vi "内部交互全局变量.vi"() -> ()   [LabVIEW 2016, in "环境动力监测库.lvlib"]
panel:
  out "监测配置输出":T1
  in  "名称或相对路径":string="data\\pem.ini"
  out "仁科通信解析":T2
  out "其他":T3 {"北斗-GPS"."GPS"."纬度:" format="%#.2g"; "北斗-GPS"."GPS"."经度:" format="%#.2g"; "北斗-GPS"."北斗"."纬度:" format="%#.2g"; "北斗-GPS"."北斗"."经度:" format="%#.2g"}
  out "安防模块":T4
  out "暖通模块":T5
  out "供电模块":T6 {"蓄电池24V"."电量" format="%.0f %"; "蓄电池24V"."电池电量:" scale=0.0..100.0; "蓄电池12V"."电量" format="%.0f %"; "蓄电池12V"."电池电量:" scale=0.0..100.0; "UPS"."电量" format="%.0f %"; "UPS"."电池电量:" scale=0.0..100.0}
  out "遥控开关机状态":bool
  out "系统参数":T7
  out "告警状态":T8
  out "传感器状态":T9
  out "运行状态":T10
  # "电源管理"
  # "GPS"
  # "北斗"
  # "真角"
  # "m/s"
  # "℃"
  # "bars"
  # "℃"
  # "℃"
  # "℃"
  # "V"
  # "V"
  # "V"
  # "V"
  # "V"
  # "V"
  # "A"
  # "V"
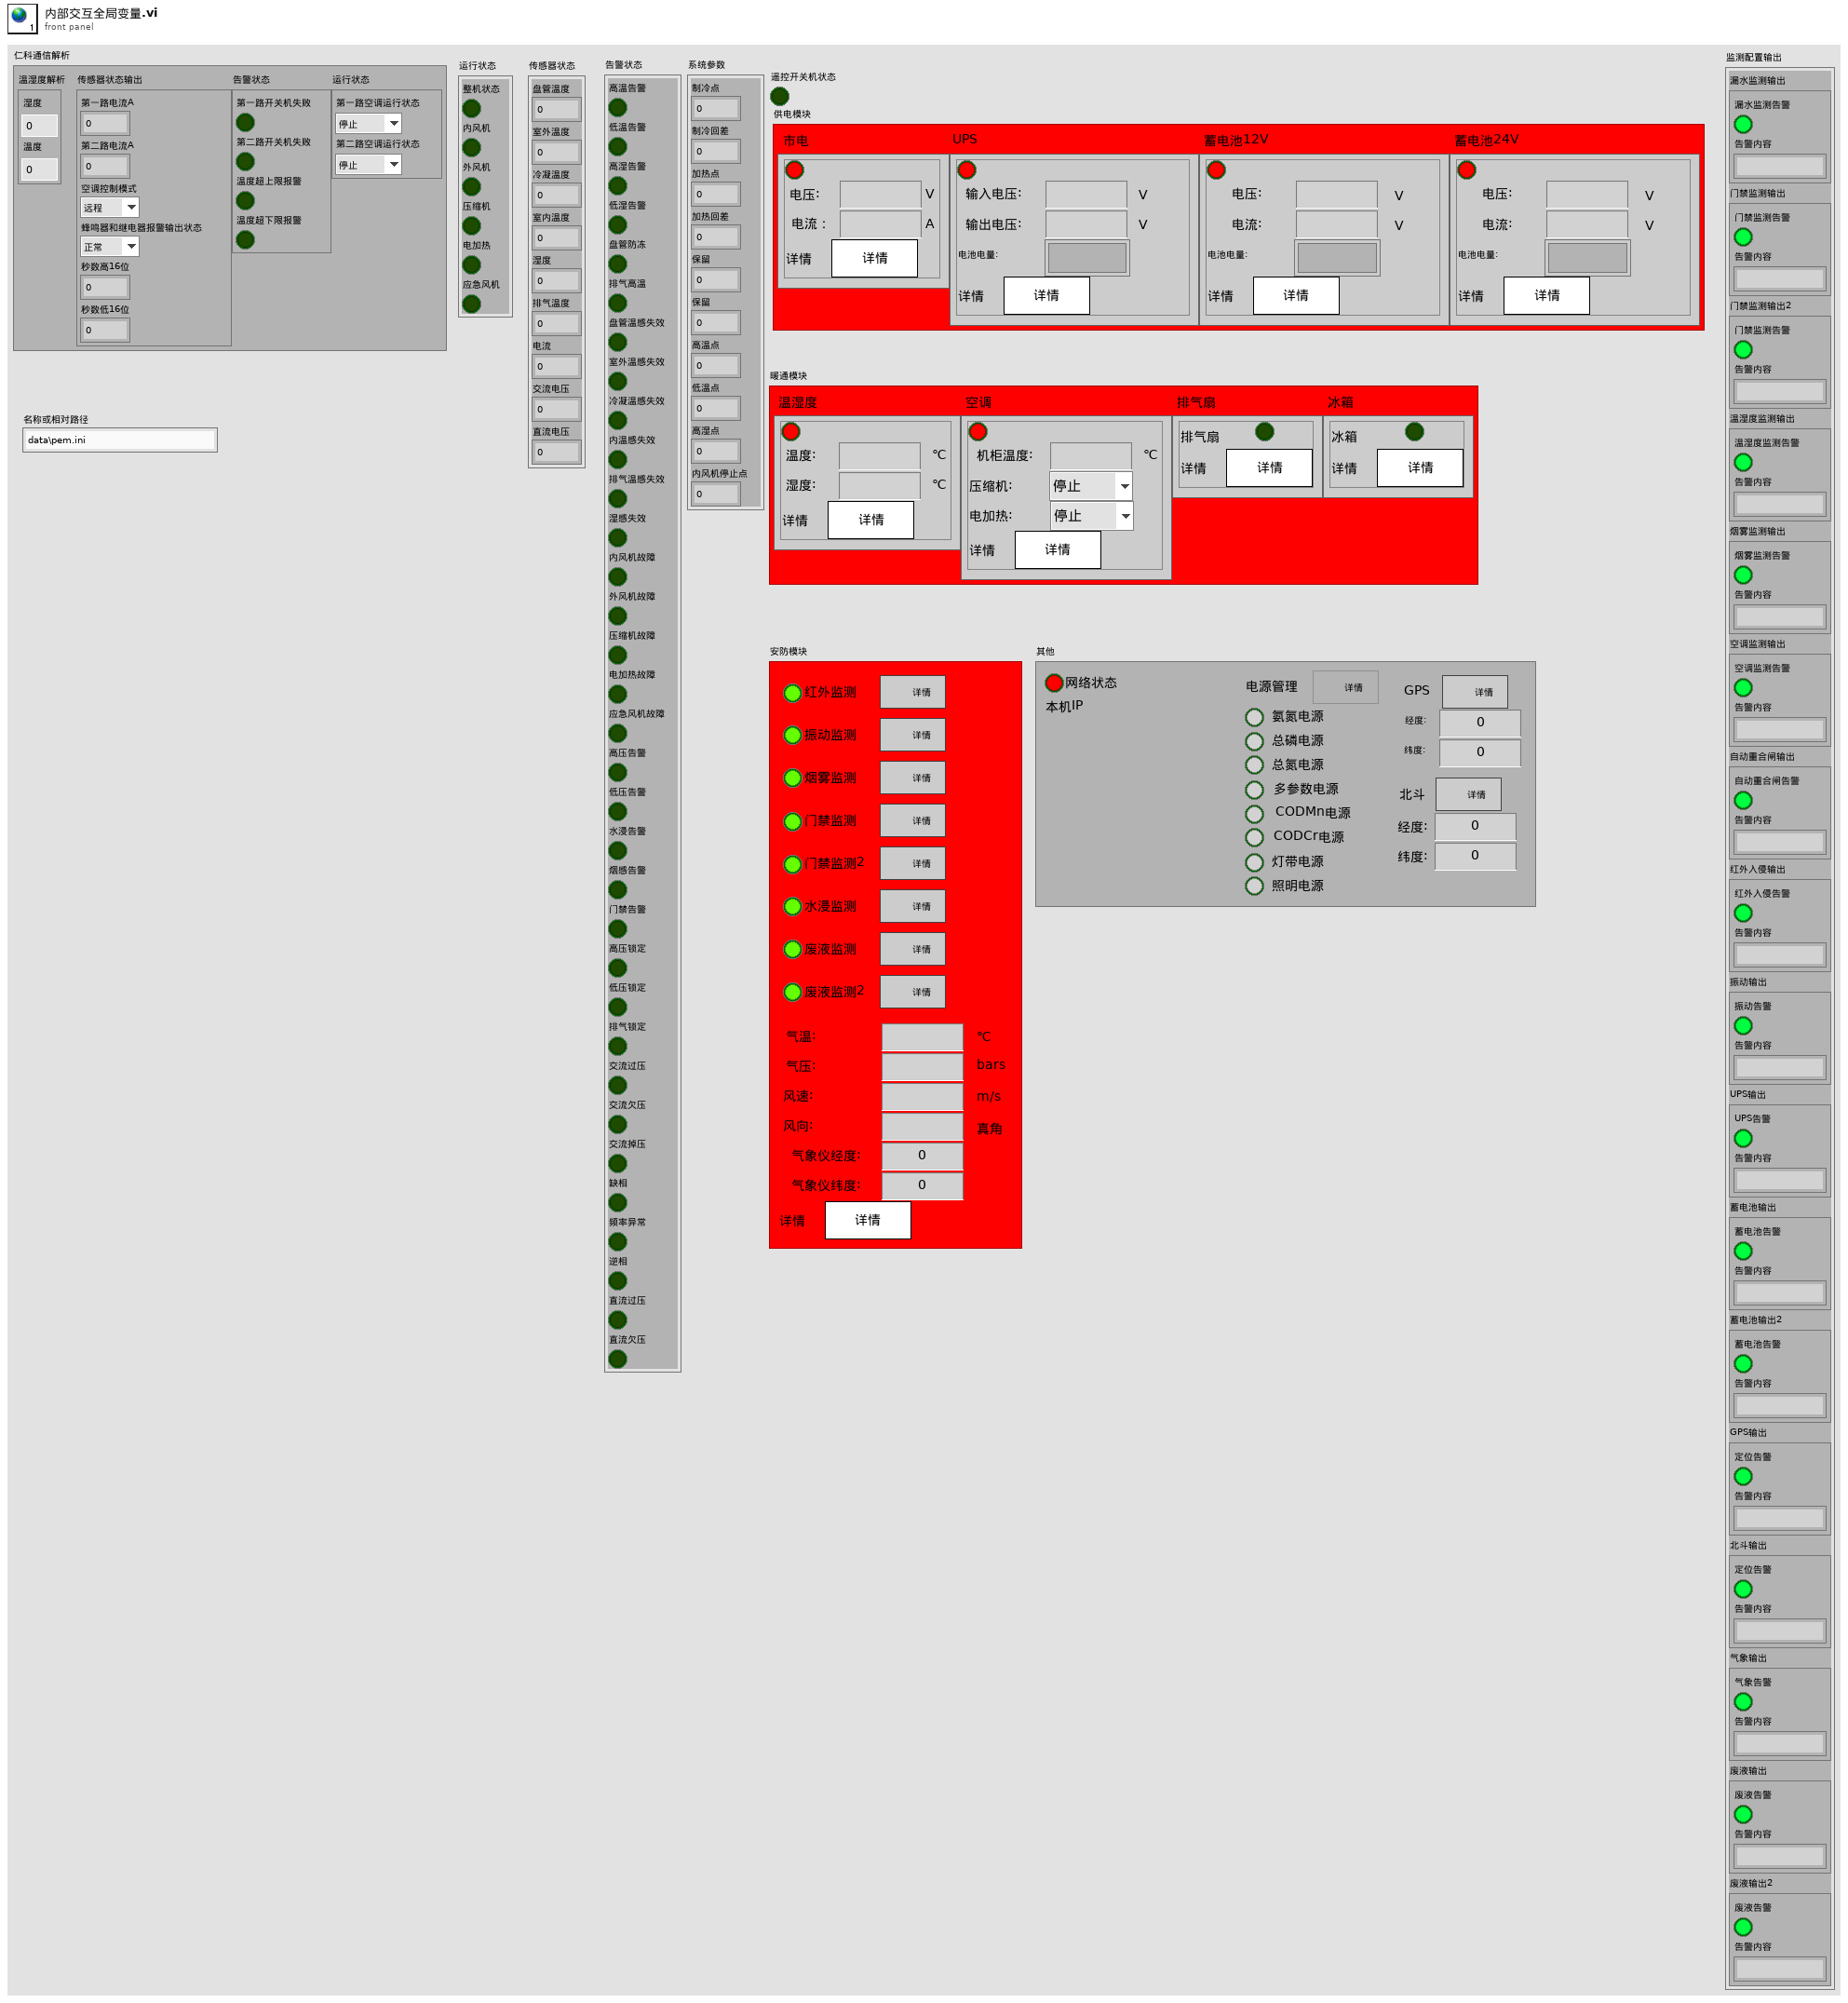
[diagram p1: front panel]
types:
  T1 = cluster{"漏水监测输出":cluster{"漏水监测告警":bool, "告警内容":string}, "门禁监测输出":cluster{"门禁监测告警":bool, "告警内容":string}, "门禁监测输出2":cluster{"门禁监测告警":bool, "告警内容":string}, "温湿度监测输出":cluster{"温湿度监测告警":bool, "告警内容":string}, "烟雾监测输出":cluster{"烟雾监测告警":bool, "告警内容":string}, "空调监测输出":cluster{"空调监测告警":bool, "告警内容":string}, "自动重合闸输出":cluster{"自动重合闸告警":bool, "告警内容":string}, "红外入侵输出":cluster{"红外入侵告警":bool, "告警内容":string}, "振动输出":cluster{"振动告警":bool, "告警内容":string}, "UPS输出":cluster{"UPS告警":bool, "告警内容":string}, "蓄电池输出":cluster{"蓄电池告警":bool, "告警内容":string}, "蓄电池输出2":cluster{"蓄电池告警":bool, "告警内容":string}, "GPS输出":cluster{"定位告警":bool, "告警内容":string}, "北斗输出":cluster{"定位告警":bool, "告警内容":string}, "气象输出":cluster{"气象告警":bool, "告警内容":string}, "废液输出":cluster{"废液告警":bool, "告警内容":string}, "废液输出2":cluster{"废液告警":bool, "告警内容":string}}
  T2 = cluster{"温湿度解析":cluster{"湿度":dbl, "温度":dbl}, "传感器状态输出":cluster{"第一路电流A":u16, "第二路电流A":u16, "空调控制模式":enum16{"远程", "自动"}, "蜂鸣器和继电器报警输出状态":enum16{"正常", "报警"}, "秒数高16位":u16, "秒数低16位":u16}, "告警状态":cluster{"第一路开关机失败":bool, "第二路开关机失败":bool, "温度超上限报警":bool, "温度超下限报警":bool}, "运行状态":cluster{"第一路空调运行状态":enum16{"停止", "制冷", "制热", "未知"}, "第二路空调运行状态":enum16{"停止", "制冷", "制热", "未知"}}}
  T3 = cluster{"网络参数":cluster{"网络状态":bool, "本机IP":string[]}, "电源管理":cluster{"电源管理":bool, "氨氮电源":bool, "总磷电源":bool, "总氮电源":bool, "多参数电源":bool, "CODMn电源":bool, "CODCr电源":bool, "灯带电源":bool, "照明电源":bool}, "北斗-GPS":cluster{"GPS":cluster{"经度:":sgl, "纬度: ":sgl, "GPS监测":bool}, "北斗":cluster{"经度:":sgl, "纬度:":sgl, "北斗监测":bool}}}
  T4 = cluster{"传感器":cluster{"红外监测":cluster{"红外监测":bool, "红外入侵监测":bool}, "振动监测":cluster{"振动监测":bool, "振动监测 2":bool}, "烟雾监测":cluster{"烟雾监测":bool, "烟雾监测 2":bool}, "门禁监测":cluster{"门禁监测":bool, "门禁开关监测":bool}, "门禁2监测":cluster{"门禁监测2":bool, "门禁开关监测2":bool}, "水浸监测":cluster{"水浸监测":bool, "漏水详情":bool}, "废液监测":cluster{"废液监测":bool, "废液详情":bool}, "废液监测2":cluster{"废液监测2":bool, "废液2详情":bool}}, "气象仪":cluster{"气温: ":sgl, "气压: ":sgl, "风速:":sgl, "风向:":sgl, "气象仪经度: ":sgl, "气象仪纬度: ":sgl, "详情  ":bool}}
  T5 = cluster{"温湿度":cluster{"状态":bool, "温度:":sgl, "湿度:":sgl, "详情  ":bool}, "空调":cluster{"状态":bool, "机柜温度:":sgl, "压缩机:":enum16{"停止", "运行"}, "电加热:":enum16{"停止", "运行"}, "详情  ":bool}, "排气扇":cluster{"排气扇":bool, "详情  ":bool}, "冰箱":cluster{"冰箱":bool, "详情  ":bool}}
  T6 = cluster{"市电":cluster{"状态":bool, "电压:":u16, "电流：":dbl, "详情  ":bool}, "UPS":cluster{"状态":bool, "输入电压:":sgl, "输出电压:":sgl, "电池电量:":u8, "电量":u16, "详情  ":bool}, "蓄电池12V":cluster{"状态":bool, "电压:":sgl, "电流:":sgl, "电池电量:":u8, "电量":u16, "详情  ":bool}, "蓄电池24V":cluster{"状态":bool, "电压:":sgl, "电流:":sgl, "电池电量:":u8, "电量":u16, "详情  ":bool}}
  T7 = cluster{"制冷点":u16, "制冷回差":u16, "加热点":u16, "加热回差":u16, "保留":u16, "保留":u16, "高温点":u16, "低温点":u16, "高湿点":u16, "内风机停止点":u16}
  T8 = cluster{"高温告警":bool, "低温告警":bool, "高湿告警":bool, "低湿告警":bool, "盘管防冻":bool, "排气高温":bool, "盘管温感失效":bool, "室外温感失效":bool, "冷凝温感失效":bool, "内温感失效":bool, "排气温感失效":bool, "湿感失效":bool, "内风机故障":bool, "外风机故障":bool, "压缩机故障":bool, "电加热故障":bool, "应急风机故障":bool, "高压告警":bool, "低压告警":bool, "水浸告警":bool, "烟感告警":bool, "门禁告警":bool, "高压锁定":bool, "低压锁定":bool, "排气锁定":bool, "交流过压":bool, "交流欠压":bool, "交流掉压":bool, "缺相":bool, "频率异常":bool, "逆相":bool, "直流过压":bool, "直流欠压":bool}
  T9 = cluster{"盘管温度":u16, "室外温度":u16, "冷凝温度":u16, "室内温度":u16, "湿度":u16, "排气温度":u16, "电流":u16, "交流电压":u16, "直流电压":u16}
  T10 = cluster{"整机状态":bool, "内风机":bool, "外风机":bool, "压缩机":bool, "电加热":bool, "应急风机":bool}
diagram:
